vi "test1.vi"() -> ()   [LabVIEW 2011]
panel:
  in  "stop":bool
  out "String 2":string
  in  "String":string="4444444"
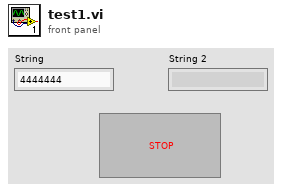
[diagram p1: front panel]
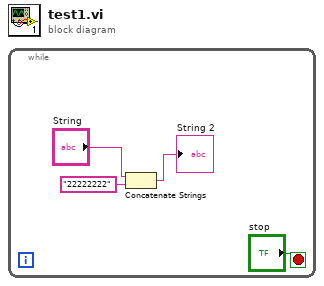
[diagram p0: block diagram]
diagram:
  n1 = while {
    stop <- "stop" stop-if-true
    n2 = Concatenate Strings("String", "22222222" ("string")) -> (→"String 2":string)
  }
